vi "GetTriggerOutputLine.vi"(8 "Error In":errorcluster, 11 "Keithley 6482 In":refnum<visa-resource-name>) -> (0 "Error Out":errorcluster, 2 "Line (1-6)":u8, 3 "Keithley 6482 Out":refnum<visa-resource-name>)   [LabVIEW 8.6, in "Keithley-6482-Visa.lvlib"]
uses:
  Keithley-6482-Visa.lvlib
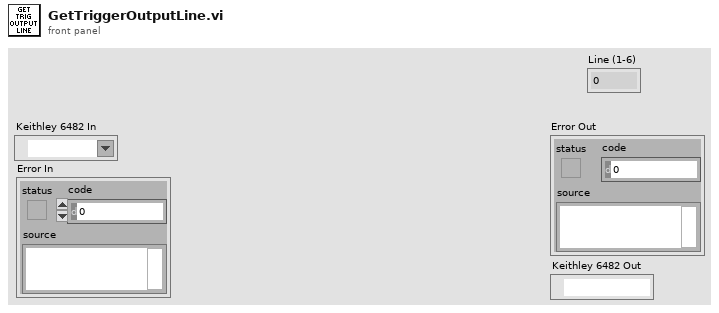
[diagram p1: front panel]
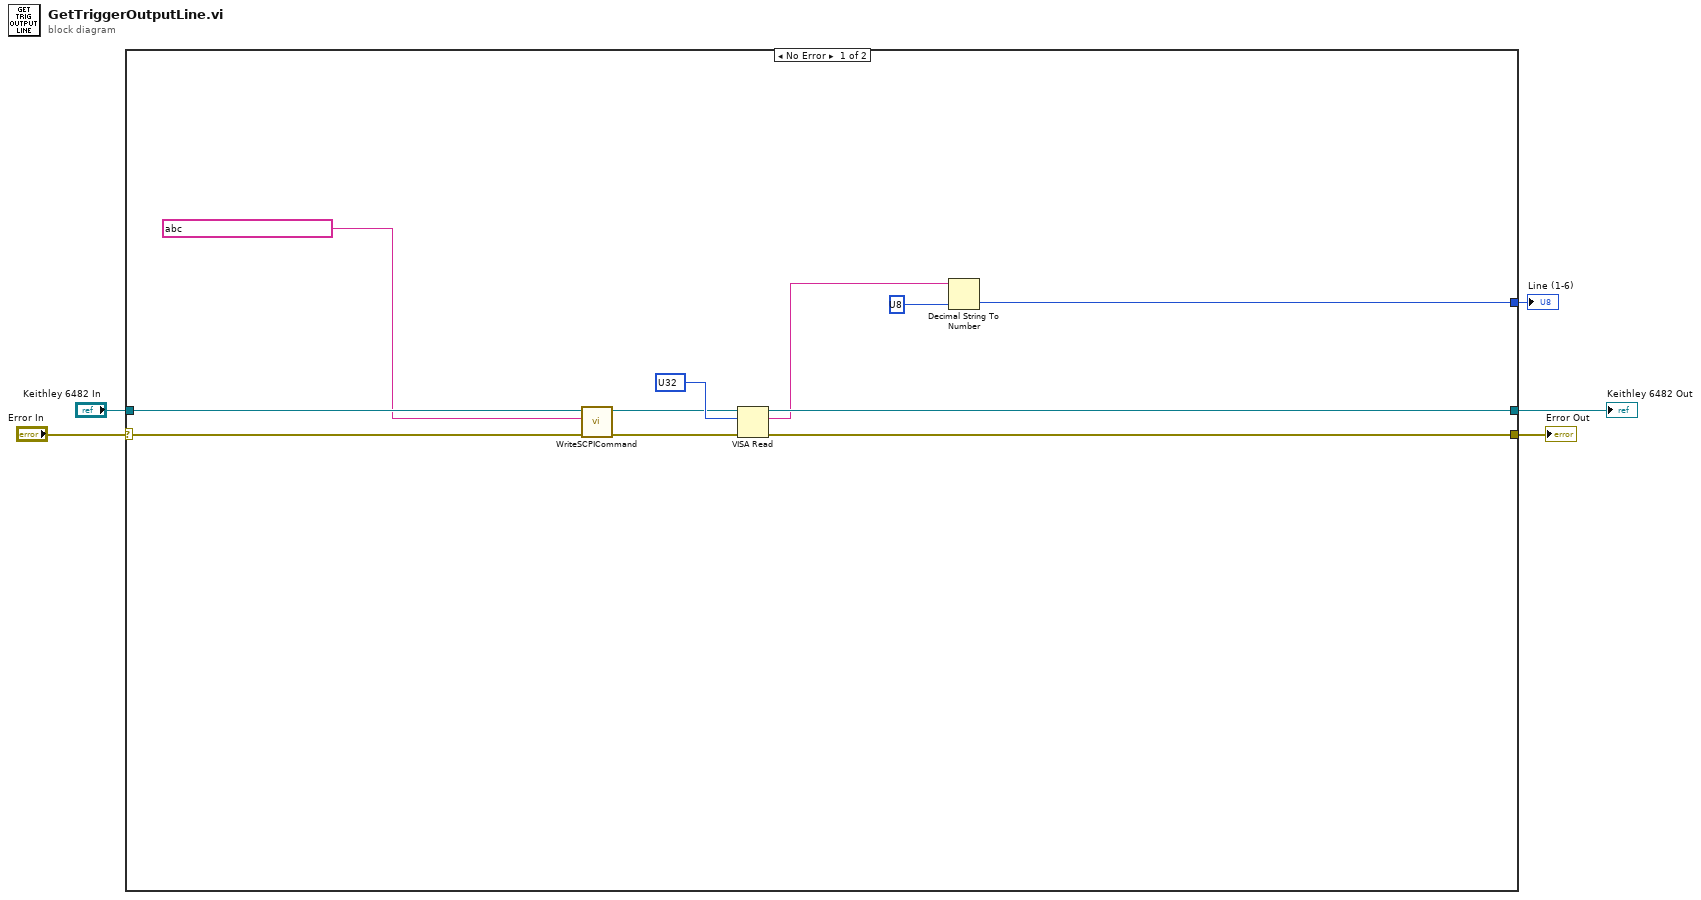
[diagram p0: block diagram]
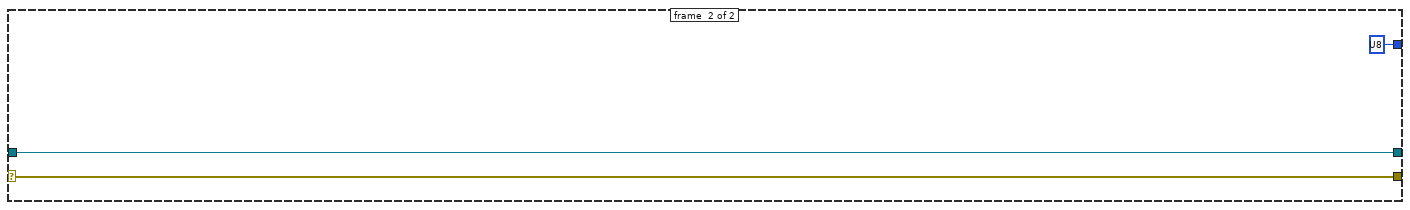
[diagram p2: hidden frame]
diagram:
  n1 = case shown="No Error" "Error In" {
    selector: "Error In" -> [w11 w18]
    tunnel: "Keithley 6482 In" -> [w10 w19]
    tunnel: [w16 w18] -> w3
    tunnel: [w15 w19] -> w2
    tunnel: [w6 u8 ?] -> w1
    frame #0 {
      n2 = call "WriteSCPICommand.vi"("Error In"=w11, "SCPI Command"=string ? ("string"), "Keithley 6482 In"=w10) -> ("Error Out"=w12:errorcluster, "Keithley 6482 Out"=w13:refnum<visa-resource-name>)  [unwired: 7 in]
      n3 = VISA Read(VISA resource name=w13, byte count=u32 ?, error in (no error)=w12) -> (VISA resource name out=w15:refnum<visa-resource-name>, read buffer=w8:string, error out=w16:errorcluster)  [unwired: 1 out]
      n4 = Decimal String To Number(string=w8, default (0L)=u8 ? ("default (0 DBL)")) -> (number=w6:u8)  [unwired: 1 in, 1 out]
    }
    frame #1 {
    }
  }
  "Error Out" <- w3
  "Keithley 6482 Out" <- w2
  "Line (1-6)" <- w1
